vi "Begin Timestamped Segment.vi"(8 "error in (no error)":errorcluster, 10 "Initial data":refnum<class "Array.lvclass">, 11 "TreeNode in":refnum<class "TreeNode.lvclass">) -> (0 "error out":errorcluster, 3 "TreeNode out":refnum<class "TreeNode.lvclass">)   [LabVIEW 2015, in "MDSplus.lvlib" / "TreeNode.lvclass"]
doc: "Begin a new data segment."
uses:
  <vilib>/MDSplus/Classes/Data_Class/TreeNode_Class/TreeNode.lvclass
  <vilib>/MDSplus/Classes/Data_Class/Array_Class/Array.lvclass
  <vilib>/MDSplus/Classes/Data_Class/Data.lvclass
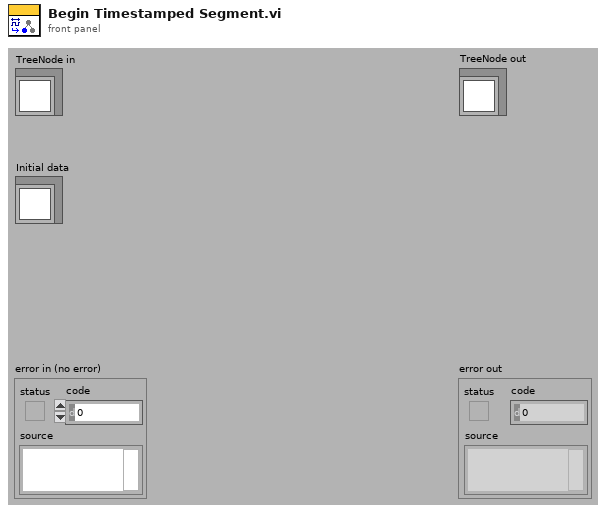
[diagram p1: front panel]
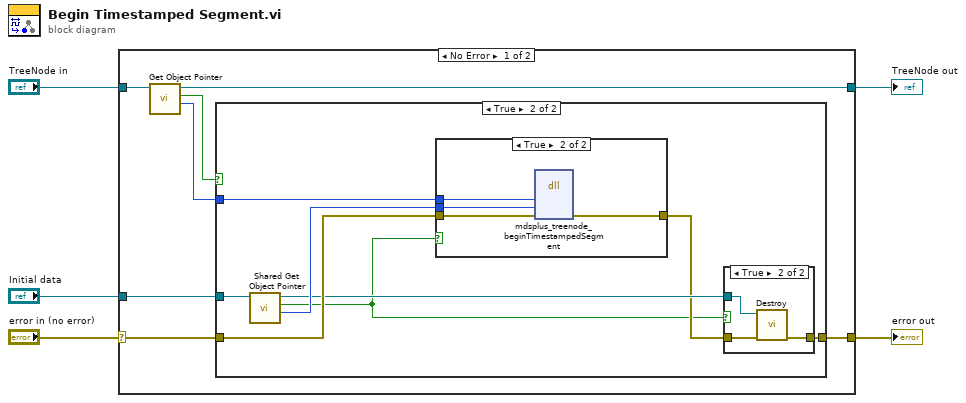
[diagram p0: block diagram]
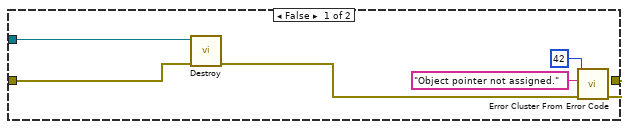
[diagram p2: hidden frame]
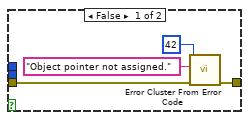
[diagram p4: hidden frame]
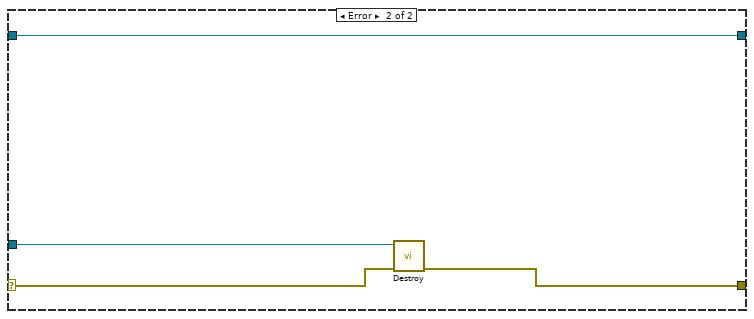
[diagram p5: hidden frame]
diagram:
  n1 = case shown="No Error" "error in (no error)" {
    selector: "error in (no error)" -> [w12 w40]
    tunnel: [w11 w39] -> w4
    tunnel: [w8 w42] -> w3
    tunnel: "TreeNode in" -> [w9 w42]
    tunnel: "Initial data" -> [w10 w41]
    frame No Error {
      n2 = call-dynamic "Get Object Pointer.vi"("Data in"=w9) -> ("Object Pointer"=w6:i64, "Assigned object pointer?"=w7:bool, "Data out"=w8:refnum<class "TreeNode.lvclass">)  [unwired: 8 in]
      n3 = case shown="True" w7 {
        tunnel: w12 -> [w18 w26]
        tunnel: [w14 w19] -> w11
        tunnel: w10 -> [w17 w25]
        tunnel: w6 -> [_ w21]
        frame False {
          n4 = call-dynamic "Destroy.vi"("error in (no error)"=w18, "Array in"=w17) -> ("error out"=w13:errorcluster)  [unwired: 9 in]
          n5 = call <vilib>:"Error Cluster From Error Code.vi"("error in (no error)"=w13, "error message (\"\")"="Object pointer not assigned." ("error message (\"\")"), "error code (0)"=42) -> ("error out"=w14:errorcluster)  [unwired: 6 in]
        }
        frame True {
          n6 = call <vilib>:"Shared Get Object Pointer.vi"("Data in"=w25) -> ("Object Pointer"=w24:i64, "Assigned object pointer?"=w20:bool, "Data out"=w23:refnum<class "Array.lvclass">)  [unwired: 8 in]
          n7 = case shown="True" w20 {
            tunnel: w26 -> [w32 w38]
            tunnel: [w31 w37] -> w22
            tunnel: w24 -> [_ w36]
            tunnel: w21 -> [_ w35]
            frame False {
              n8 = call <vilib>:"Error Cluster From Error Code.vi"("error in (no error)"=w32, "error message (\"\")"="Object pointer not assigned." ("error message (\"\")"), "error code (0)"=42) -> ("error out"=w31:errorcluster)  [unwired: 6 in]
            }
            frame True {
              n9 = dll-call lib="MDSobjectsLVShr" fn="mdsplus_treenode_beginTimestampedSegment"("lvTreeNodePtr"=w35, "lvInitDataPtrIn"=w36, "error"=w38) -> ("error"=w37:errorcluster)  [unwired: 6 in, 2 out]
            }
          }
          n10 = case shown="True" w20 {
            tunnel: w22 -> [w27 w30]
            tunnel: w23 -> [_ w29]
            tunnel: [w27 w28] -> w19
            frame False {
            }
            frame True {
              n11 = call-dynamic "Destroy.vi"("error in (no error)"=w30, "Array in"=w29) -> ("error out"=w28:errorcluster)  [unwired: 9 in]
            }
          }
        }
      }
    }
    frame Error {
      n12 = call-dynamic "Destroy.vi"("error in (no error)"=w40, "Array in"=w41) -> ("error out"=w39:errorcluster)  [unwired: 9 in]
    }
  }
  "error out" <- w4
  "TreeNode out" <- w3
